vi "shifter.vi"(4 "Read Count":u32=64, 9 "Stop":bool) -> (6 "Log":string)   [LabVIEW 2025]
uses:
  Program Files (x86)/National Instruments/LabVIEW 2025/examples/Instrument IO/Serial/support/Serial - ASCII Characters.ctl
  <vilib>/Utility/error.llb/Trim Whitespace One-Sided.vi
  <vilib>/Instr/_visa.llb/VISA Configure Serial Port (Instr).vi
  <vilib>/regexp/Match Regular Expression.xnode
panel:
  out "Torque/MPH":cluster{dbl[], dbl[]}[](graph)
  out "OPTIMAL\nGEAR":i8=1
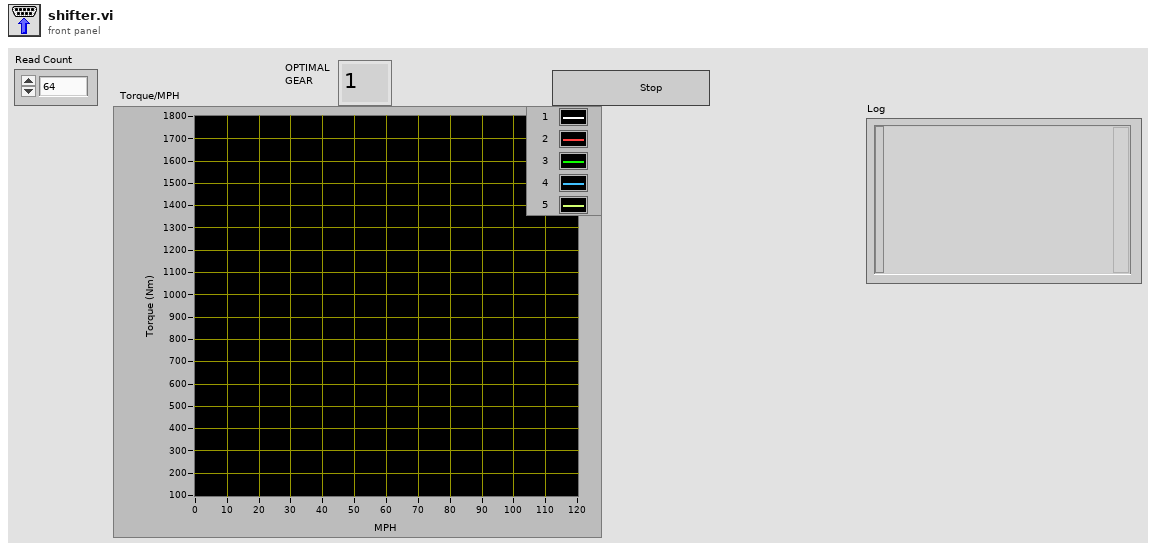
[diagram p1: front panel]
types:
  T1 = typedef "Serial - ASCII Characters.ctl" = enum16{"NUL", "SOH", "STX", "ETX", "EOT", "ENQ", "ACK", "BEL", "BS", "HT", "LF", "VT", "FF", "CR", "SO", "SI", "DLE", "DC1", "DC2", "DC3", "DC4", "NAK", "SYN", "ETB", "CAN", "EM", "SUB", "ESC", "FS", "GS", "RS", "US", "SP", "!", "\"", "#", "$", "%", "&", "'", "(", ")", "*", "+", ",", "- (-)", ".", "/", "0", "1", "2", "3", "4", "5", "6", "7", "8", "9", ":", ";", "<", "=", ">", "?", "@", "A", "B", "C", "D", "E", "F", "G", "H", "I", "J", "K", "L", "M", "N", "O", "P", "Q", "R", "S", "T", "U", "V", "W", "X", "Y", "Z", "[", "\\", "]", "^", "_", "`", "a", "b", "c", "d", "e", "f", "g", "h", "i", "j", "k", "l", "m", "n", "o", "p", "q", "r", "s", "t", "u", "v", "w", "x", "y", "z", "{", "|", "}", "~"}
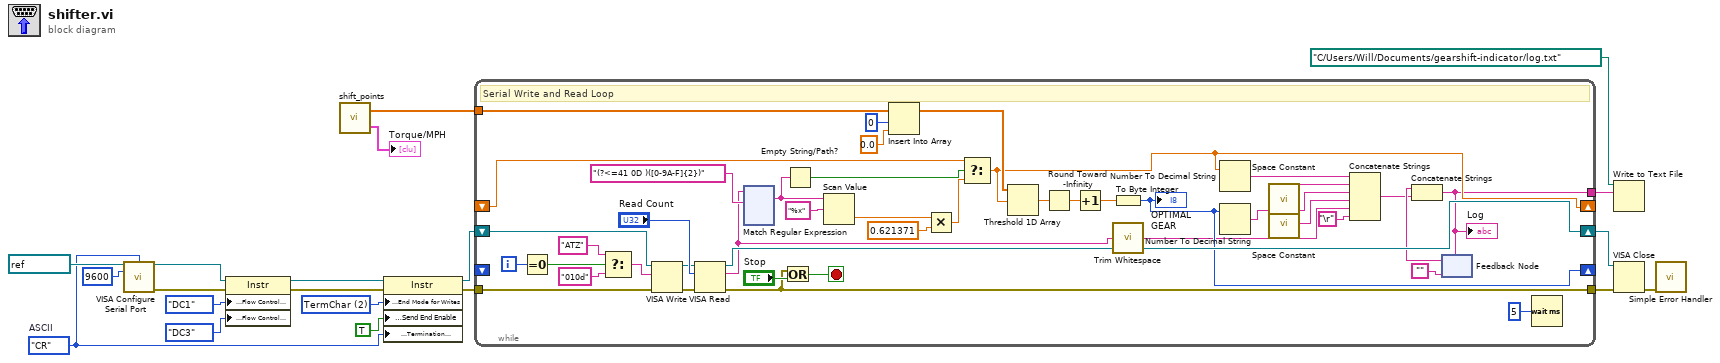
[diagram p0: block diagram]
diagram:
  w5 = Serial_-_ASCII_Characters."CR"  # ASCII
  w18 = u16 2 items=["None", "LastBit", "TermChar", "Break"] ("Serial Settings:Serial End Mode for Writes")
  n1 = call-poly "VISA Configure Serial Port"("VISA resource name"=refnum<visa-resource-name> "COM9", "termination char\n(0xA = '\\n' = LF)"=w5, "baud rate (9600)"=u32 9600) -> ("VISA resource name out"=w11:refnum<visa-resource-name>, "error out"=w7:errorcluster)  [unwired: 11 in]
  n2 = property class="Instr"(reference=w11, error in=w7, "Serial Settings:Flow Control XON Character"=Serial_-_ASCII_Characters."DC1" ("XOFF"), "Serial Settings:Flow Control XOFF Character"=Serial_-_ASCII_Characters."DC3" ("XOFF")) -> (reference out=w10:refnum<visa-resource-name>, error out=w6:errorcluster)
  n3 = call "shift_points.vi"() -> ("Torque/MPH"=→"Torque/MPH":cluster{dbl[], dbl[]}[], "Intercepts"=w2:dbl[])  [unwired: 2 in]
  n4 = property class="Instr"(reference=w10, error in=w6, "Serial Settings:End Mode for Writes"=w18, "Message Based Settings:Send End Enable"=TRUE, "Message Based Settings:Termination Character"=w5) -> (reference out=w16:refnum<visa-resource-name>, error out=w15:errorcluster)
  n5 = while {
    shift-right: [w59] -> w13
    shift-left: w16 -> [w61]
    tunnel: w15 -> [w60]
    tunnel: [w58] -> w12
    shift-right: [w38] -> _
    shift-left: _ -> [_]
    shift-right: [w30] -> _
    shift-left: _ -> [w29]
    tunnel: [w22] -> w3
    tunnel: w2 -> [w21]
    i -> [w57]
    stop <- w47 stop-if-true
    # "Serial Write and Read Loop"
    n6 = Equal To 0?(x=w57) -> (x = 0?=w56:bool)
    n7 = Select(t="ATZ", s=w56, f="010d" ("Command")) -> (s? t:f=w53:string)
    n8 = VISA Write(VISA resource name=w61, write buffer=w53, error in (no error)=w60) -> (VISA resource name out=w34:refnum<visa-resource-name>, error out=w33:errorcluster)  [unwired: 1 out]
    n9 = VISA Read(VISA resource name=w34, byte count="Read Count", error in (no error)=w33) -> (VISA resource name out=w59:refnum<visa-resource-name>, read buffer=w35:string, error out=w58:errorcluster)  [unwired: 1 out]
    n10 = xnode "Match Regular Expression"("input string"=w35, "regular expression"="(?<=41 0D )([0-9A-F]{2})") -> ("whole match"=w32:string)  [unwired: 4 in, 4 out]
    n11 = Or(x=w58, y="Stop") -> (x .or. y?=w47:bool)
    n12 = Empty String/Path?(string/path=w32) -> (empty?=w31:bool)
    n13 = Scan Value(string=w32, format string="%x") -> (value=w28:dbl)  [unwired: 1 in, 1 out]
    n14 = Insert Into Array(array=w21, index=0, new element=0.0 ("new element/subarray")) -> (w41:dbl[])
    n15 = Multiply(x=w28, y=0.621371) -> (x*y=w26:dbl)
    n16 = Select(t=w29, s=w31, f=w26) -> (s? t:f=w30:dbl)
    n17 = Threshold 1D Array(2:w30, 3:w41) -> (0:w44:dbl)  [unwired: 1 in]
    n18 = Round Toward -Infinity(1:w44) -> (0:w43:dbl)
    n19 = Increment(x=w43) -> (x+1=w42:dbl)
    n20 = To Byte Integer(number=w42) -> (8bit integer=w38:i8)
    "OPTIMAL\nGEAR" <- w38
    n21 = call <vilib>:"Trim Whitespace.vi"("string"=w35) -> ("trimmed string"=w23:string)  [unwired: 1 in]
    n22 = Number To Decimal String(number=w30) -> (decimal integer string=w40:string)  [unwired: 1 in]
    n23 = Number To Decimal String(number=w38) -> (decimal integer string=w37:string)  [unwired: 1 in]
    n24 = call <vilib>:"Space Constant.vi"() -> ("String"=w36:string)
    n25 = call <vilib>:"Space Constant.vi"() -> ("String"=w24:string)
    n26 = Concatenate Strings(w40, w36, w37, w24, w23, "\r") -> (w39:string)
    n27 = feedback #1("") -> (w49:string)
    n28 = Concatenate Strings(w49, w39) -> (w22:string)
    "Log" <- w22
    n29 = feedback-in #1(w22) -> ()
    n30 = Wait (ms)(milliseconds to wait=u32 5) -> ()  [unwired: 1 out]
  }
  n31 = Write to Text File(file (use dialog)=path "C:/Users/Will/Documents/gearshift-indicator/log.txt", text=w3) -> ()  [unwired: 2 in, 3 out]
  n32 = VISA Close(VISA resource name=w13, error in (no error)=w12) -> (error out=w14:errorcluster)
  n33 = call <vilib>:"Simple Error Handler.vi"("error in (no error)"=w14) -> ()  [unwired: 1 in, 8 out]
